vi "Find First Matching Resource (String).vi"(6 "Error if not found? (F)":bool, 8 "Error in":errorcluster caption="Error in (no error)", 10 "Resource Types":string[](array[string]), 11 "Resources":T1) -> (0 "Error out":errorcluster, 1 "Index":i32, 2 "Found?":bool, 3 "Resource":T2)   [LabVIEW 2018, in "Resource Manipulation.lvlib"]
uses:
  Resource Manipulation.lvlib
  Resource.ctl
  Resource Array.ctl
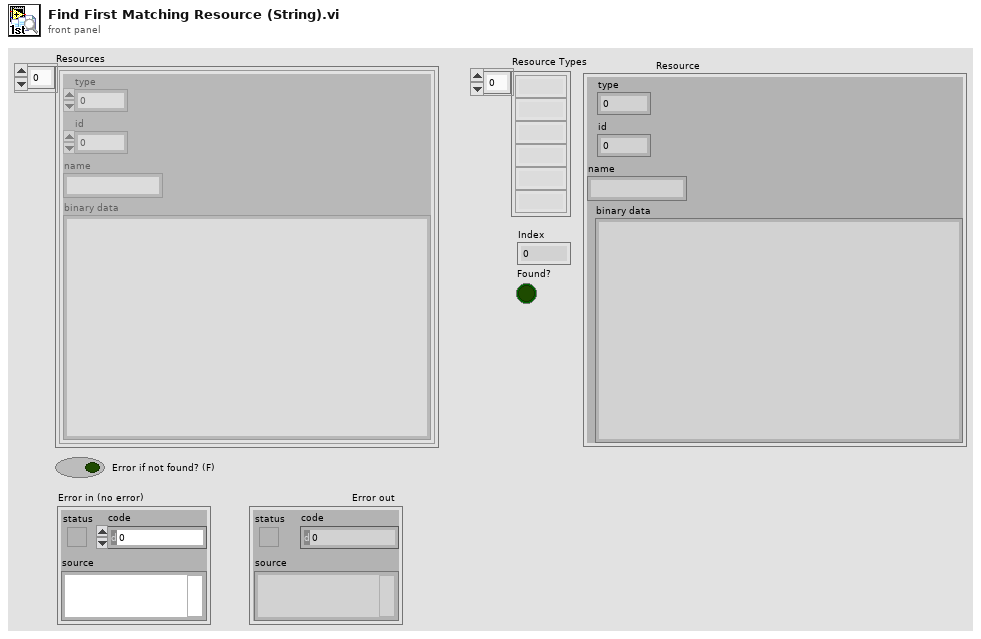
[diagram p1: front panel]
types:
  T1 = typedef "Resource Manipulation.lvlib/Resource Array.ctl" = T2[]
  T2 = typedef "Resource Manipulation.lvlib/Resource.ctl" = cluster{"type":u32, "id":i32, "name":string, "binary data":string}
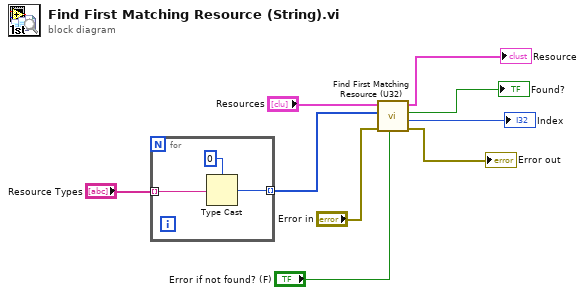
[diagram p0: block diagram]
diagram:
  n1 = for {
    tunnel: "Resource Types" -> [w11] mode=indexing
    tunnel: [w10] -> w7 mode=indexing
    n2 = Type Cast(type=u32 0, x=w11) -> (*(type *) &x=w10:u32)
  }
  n3 = call "Find First Matching Resource (U32).vi"("Error if not found? (F)"="Error if not found? (F)", "Error in"="Error in", "Resource Types"=w7, "Resources"="Resources") -> ("Error out"=→"Error out":errorcluster, "Index"=→"Index":i32, "Found?"=→"Found?":bool, "Resource"=→"Resource":T2)  [unwired: 4 in]
